vi "publish -- get frequency and voltage.vi"(0 "running lorentzian in":T1={"A (VHz)"=-1.0311345636926572, "ω (Hz)"=-1.0311345636926572, "Γ (Hz)"=-1.0311345636926572, "φ (rad)"=-1.0311345636926572, "Q"=-1.0311345636926572, "Norm  Ampl"=-1.0311345636926572, "z∞ (V)"=-1.0311345636926572+0.0i, "4corners"={"z (-pi/2)"=-1.0311345636926572+0.5736824521422934i, "z(inf)"=-0.5200164984937075+1.0975277942502903i, "z (pi/2)"=-1.0311345636926572+0.5736824521422934i, "z center"=-0.5136528600391839+0.580046090596817i, "z(0)"=-0.5200164984937075+1.0975277942502903i, "radius"=-1.0311345636926572}} {"z∞ (V)" format="%#_4p"; "Q" format="%#_4p"; "φ (rad)" format="%#_3p"; "Γ (Hz)" format="%#_5p"; "ω (Hz)" format="%#_9p"; "A (VHz)" format="%#_3p"}, 1 "publisher action":T3, 5 "freq IN (Hz)":dbl=1000.0 format="%#_10f", 7 "static lorentzian IN":T1={"A (VHz)"=-1.0311345636926572, "ω (Hz)"=-1.0311345636926572, "Γ (Hz)"=-1.0311345636926572, "φ (rad)"=-1.0311345636926572, "Q"=-1.0311345636926572, "Norm  Ampl"=-1.0311345636926572, "z∞ (V)"=-1.0311345636926572+0.0i, "4corners"={"z (-pi/2)"=-1.0311345636926572+0.5736824521422934i, "z(inf)"=-0.5200164984937075+1.0975277942502903i, "z (pi/2)"=-1.0311345636926572+0.5736824521422934i, "z center"=-0.5136528600391839+0.580046090596817i, "z(0)"=-0.5200164984937075+1.0975277942502903i, "radius"=-1.0311345636926572}} {"z∞ (V)" format="%#_4p"; "Q" format="%#_4p"; "φ (rad)" format="%#_3p"; "Γ (Hz)" format="%#_5p"; "ω (Hz)" format="%#_9p"; "A (VHz)" format="%#_3p"}, 9 "Voltage IN (V)":cdb=1.133070214302279+0.0i, 11 "gamma IN (Hz)":dbl=1000.0) -> (4 "running lorentzian out":T1={"A (VHz)"=-1.0311345636926572, "ω (Hz)"=-1.0311345636926572, "Γ (Hz)"=-1.0311345636926572, "φ (rad)"=-1.0311345636926572, "Q"=-1.0311345636926572, "Norm  Ampl"=-1.0311345636926572, "z∞ (V)"=-1.0311345636926572+0.0i, "4corners"={"z (-pi/2)"=-1.0311345636926572+0.5736824521422934i, "z(inf)"=-0.5200164984937075+1.0975277942502903i, "z (pi/2)"=-1.0311345636926572+0.5736824521422934i, "z center"=-0.5136528600391839+0.580046090596817i, "z(0)"=-0.5200164984937075+1.0975277942502903i, "radius"=-1.0311345636926572}} {"z∞ (V)" format="%#_4p"; "Q" format="%#_4p"; "φ (rad)" format="%#_3p"; "Γ (Hz)" format="%#_5p"; "ω (Hz)" format="%#_9p"; "A (VHz)" format="%#_3p"}, 6 "freq out (Hz)":dbl=1000.0 format="%#_10f", 8 "static lorentzian out":T1={"A (VHz)"=-1.0311345636926572, "ω (Hz)"=-1.0311345636926572, "Γ (Hz)"=-1.0311345636926572, "φ (rad)"=-1.0311345636926572, "Q"=-1.0311345636926572, "Norm  Ampl"=-1.0311345636926572, "z∞ (V)"=-1.0311345636926572+0.0i, "4corners"={"z (-pi/2)"=-1.0311345636926572+0.5736824521422934i, "z(inf)"=-0.5200164984937075+1.0975277942502903i, "z (pi/2)"=-1.0311345636926572+0.5736824521422934i, "z center"=-0.5136528600391839+0.580046090596817i, "z(0)"=-0.5200164984937075+1.0975277942502903i, "radius"=-1.0311345636926572}} {"z∞ (V)" format="%#_4p"; "Q" format="%#_4p"; "φ (rad)" format="%#_3p"; "Γ (Hz)" format="%#_5p"; "ω (Hz)" format="%#_9p"; "A (VHz)" format="%#_3p"}, 10 "Voltage out (V)":cdb=1.133070214302279+0.0i, 15 "gamma OUT (Hz)":dbl=1000.0)   [LabVIEW 2021]
uses:
  publisher action.ctl
  lorentzian.ctl
  circle corners.ctl
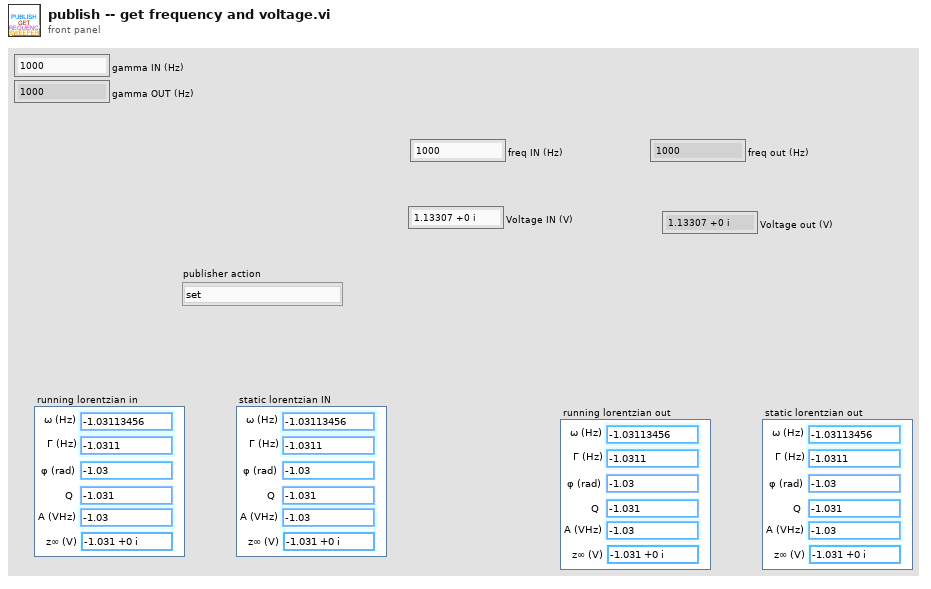
[diagram p1: front panel]
types:
  T1 = typedef "lorentzian.ctl" = cluster{"A (VHz)":dbl, "ω (Hz)":dbl, "Γ (Hz)":dbl, "φ (rad)":dbl, "Q":dbl, "Norm  Ampl":dbl, "z∞ (V)":cdb, "4corners":T2}
  T2 = typedef "circle corners.ctl" = cluster{"z (-pi/2)":cdb, "z(inf)":cdb, "z (pi/2)":cdb, "z center":cdb, "z(0)":cdb, "radius":dbl}
  T3 = typedef "publisher action.ctl" = enum16{"set", "get", "init", "check"}
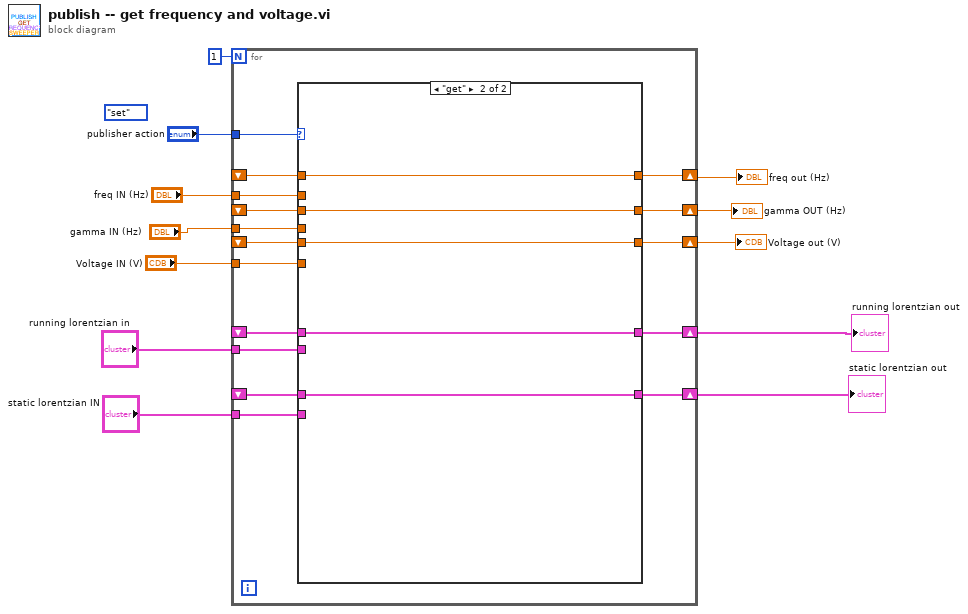
[diagram p0: block diagram]
diagram:
  (unwired) publisher_action."set" ("publisher action")
  n1 = for {
    N: 1 -> [_]
    tunnel: "publisher action" -> [w28]
    tunnel: "freq IN (Hz)" -> [w26]
    shift-right: [w27] -> w8
    shift-left: _ -> [w25]
    shift-right: [w24] -> w7
    shift-left: _ -> [w22]
    tunnel: "Voltage IN (V)" -> [w23]
    tunnel: "gamma IN (Hz)" -> [w21]
    shift-right: [w20] -> w5
    shift-left: _ -> [w19]
    tunnel: "static lorentzian IN" -> [w17]
    shift-right: [w18] -> w4
    shift-left: _ -> [w13]
    tunnel: "running lorentzian in" -> [w15]
    shift-right: [w16] -> w2
    shift-left: _ -> [w14]
    n2 = case shown="\"get\"" w28 {
      tunnel: [w33 w38] -> w27
      tunnel: w26 -> [w33 _]
      tunnel: w25 -> [_ w38]
      tunnel: [w32 w37] -> w24
      tunnel: w23 -> [w32 _]
      tunnel: w22 -> [_ w37]
      tunnel: w21 -> [w31 _]
      tunnel: [w31 w36] -> w20
      tunnel: w19 -> [_ w36]
      tunnel: [w30 w34] -> w18
      tunnel: w17 -> [w30 _]
      tunnel: [w29 w35] -> w16
      tunnel: w15 -> [w29 _]
      tunnel: w14 -> [_ w35]
      tunnel: w13 -> [_ w34]
      frame "set", Default {
      }
      frame "get" {
      }
    }
  }
  "Voltage out (V)" <- w7
  "freq out (Hz)" <- w8
  "gamma OUT (Hz)" <- w5
  "running lorentzian out" <- w2
  "static lorentzian out" <- w4
